vi "Deadband.vi"(8 "Rescaling On?":bool, 10 "Deadband Info":T1, 11 "Robot Velocities":T2) -> (2 "Sending Input?":bool, 3 "Adjusted Robot Velocities":T2)   [LabVIEW 2020]
uses:
  swerve/Type Definitions/Data/Robot Velocities.ctl
  <vilib>/Analysis/_algsub.llb/Real Vector Norm.vi
  <vilib>/Analysis/NI_AALPro.lvlib
  <vilib>/ptbypt/NI_PtbyPt.lvlib
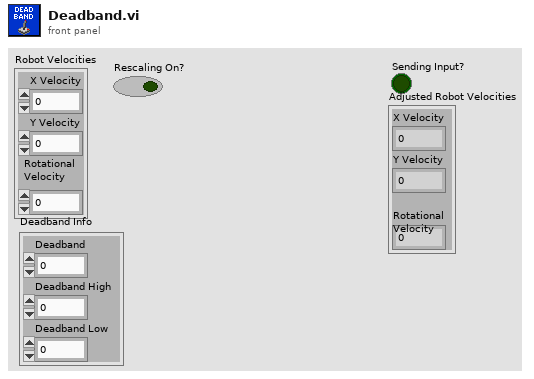
[diagram p1: front panel]
types:
  T1 = cluster{"Deadband":dbl, "Deadband High":dbl, "Deadband Low":dbl}
  T2 = typedef "Robot Velocities.ctl" = cluster{"X Velocity":dbl, "Y Velocity":dbl, "Rotational \nVelocity":dbl}
  T3 = cluster{"X Velocity":bool, "Y Velocity":bool, "Rotational \nVelocity":bool}
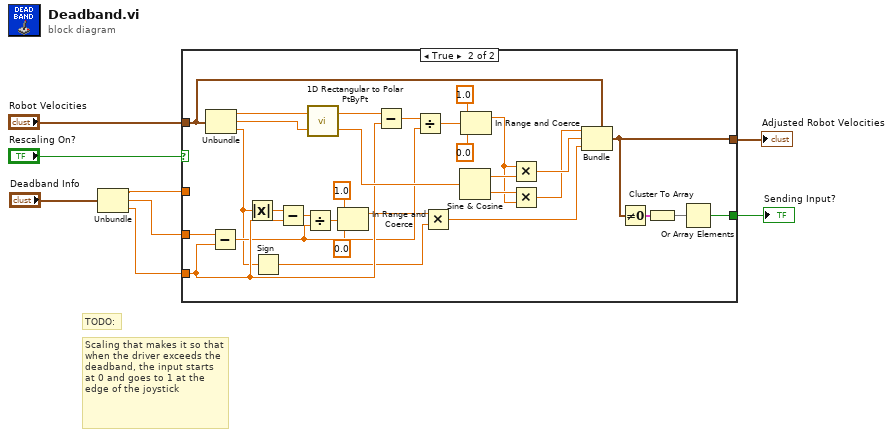
[diagram p0: block diagram]
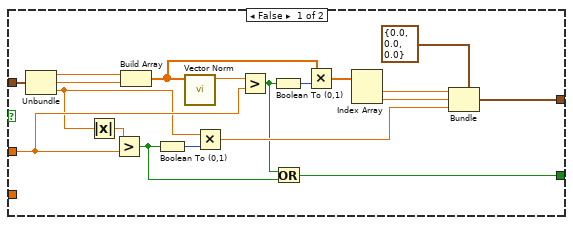
[diagram p2: hidden frame]
diagram:
  # "TODO:"
  # "Scaling that makes it so that when the driver exceeds the deadband, the input starts at 0 and goes to 1 at the edge of the joystick"
  n1 = Unbundle("Deadband Info") -> ("Deadband"=w3:dbl, "Deadband High"=w2:dbl, "Deadband Low"=w1:dbl)
  n2 = case shown="True" "Rescaling On?" {
    tunnel: "Robot Velocities" -> [w27 w45]
    tunnel: [w22 w36] -> w7
    tunnel: w3 -> [w17 _]
    tunnel: w2 -> [_ w57]
    tunnel: w1 -> [_ w42]
    tunnel: [w9 w33] -> w5
    frame False {
      n3 = Unbundle(w27) -> ("X Velocity"=w26:dbl, "Y Velocity"=w25:dbl, "Rotational \nVelocity"=w11:dbl)
      n4 = Absolute Value(x=w11) -> (abs(x)=w10:dbl)
      n5 = Greater?(x=w10, y=w17) -> (0:w23:bool)
      n6 = Build Array(w26, w25) -> (w18:dbl[])
      n7 = Boolean To (0,1)(Boolean=w23) -> (0, 1=w24:i16)
      n8 = call-poly <vilib>:"Vector Norm.vi"("Input Vector"=w18) -> ("norm"=w20:dbl)  [unwired: 9 in, 1 out]
      n9 = Multiply(x=w11, y=w24) -> (x*y=w13:dbl)
      n10 = Greater?(x=w20, y=w17) -> (0:w12:bool)
      n11 = Boolean To (0,1)(Boolean=w12) -> (0, 1=w19:i16)
      n12 = Or(x=w12, y=w23) -> (x .or. y?=w9:bool)
      n13 = Multiply(x=w18, y=w19) -> (x*y=w16:dbl[])
      n14 = Index Array(array=w16) -> (element #1=w15:dbl, element #2=w14:dbl)  [unwired: 2 in]
      n15 = Bundle(cluster=T2 {"X Velocity"=0.0, "Y Velocity"=0.0, "Rotational \nVelocity"=0.0} ("Adjusted Robot Velocities"), "X Velocity"=w15, "Y Velocity"=w14, "Rotational \nVelocity"=w13) -> (w22:T2)
    }
    frame True {
      n16 = Unbundle(w45) -> ("X Velocity"=w52:dbl, "Y Velocity"=w51:dbl, "Rotational \nVelocity"=w31:dbl)
      n17 = Subtract(x=w57, y=w42) -> (x-y=w40:dbl)
      n18 = Absolute Value(x=w31) -> (abs(x)=w32:dbl)
      n19 = Sign(1:w31) -> (0:w29:dbl)
      n20 = Subtract(x=w32, y=w42) -> (x-y=w41:dbl)
      n21 = Divide(x=w41, y=w40) -> (x/y=w37:dbl)
      n22 = call <vilib>:"1D Rectangular to Polar PtByPt.vi"("y"=w51, "x"=w52) -> ("phase"=w49:dbl, "magnitude"=w50:dbl)
      n23 = In Range and Coerce(upper limit=1.0, x=w37, lower limit=0.0) -> (coerced(x)=w30:dbl)  [unwired: 1 out]
      n24 = Subtract(x=w50, y=w42) -> (x-y=w56:dbl)
      n25 = Divide(x=w56, y=w40) -> (x/y=w55:dbl)
      n26 = Multiply(x=w30, y=w29) -> (x*y=w28:dbl)
      n27 = Sine & Cosine(0:w49) -> (1:w48:dbl, 2:w47:dbl)
      n28 = In Range and Coerce(upper limit=1.0, x=w55, lower limit=0.0) -> (coerced(x)=w46:dbl)  [unwired: 1 out]
      n29 = Multiply(x=w46, y=w48) -> (x*y=w44:dbl)
      n30 = Multiply(x=w47, y=w46) -> (x*y=w43:dbl)
      n31 = Bundle(cluster=w45, "X Velocity"=w43, "Y Velocity"=w44, "Rotational \nVelocity"=w28) -> (w36:T2)
      n32 = Not Equal To 0?(x=w36) -> (x != 0?=w35:T3)
      n33 = Cluster To Array(cluster=w35) -> (array=w34:bool[])
      n34 = Or Array Elements(Boolean array=w34) -> (logical OR=w33:bool)
    }
  }
  "Adjusted Robot Velocities" <- w7
  "Sending Input?" <- w5
